vi "oax_GS Level Measurement.vi"(0 "scaled signals [EU]":waveform(dbl)[](array[waveform]), 5 "Start":dbl, 7 "Duration":dbl, 9 "select channel":u16, 11 "error in (no error)":errorcluster) -> (4 "Peak level [EU]":dbl, 6 "RMS level [EU]":dbl, 8 "vibration signals":waveform(dbl), 15 "error out":errorcluster)   [LabVIEW 2017]
uses:
  <vilib>/addons/Sound and Vibration/svt_Level/SVL Peak Level (1 Ch).vi
  <vilib>/addons/Sound and Vibration/svt_Level/SVL RMS Level (1 Ch).vi
  <vilib>/Waveform/WDTOps.llb/WDT Get Waveform Subset DBL (LV80).vi
  <vilib>/addons/Sound and Vibration/svt_Level/SoundVib_VibrationLevel.lvlib
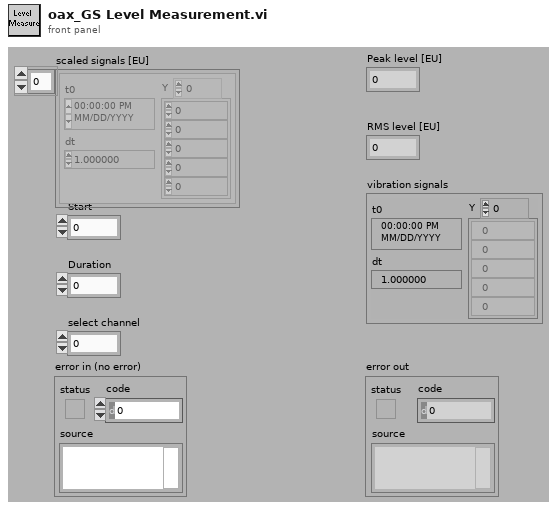
[diagram p1: front panel]
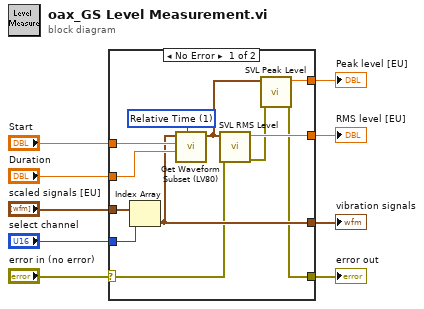
[diagram p0: block diagram]
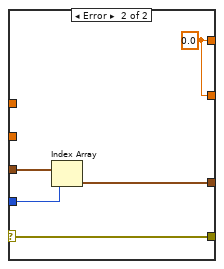
[diagram p2: hidden frame]
diagram:
  n1 = case shown="No Error" "error in (no error)" {
    selector: "error in (no error)" -> [w12 w26]
    tunnel: [w21 w25] -> w9
    tunnel: "Duration" -> [w19 _]
    tunnel: "Start" -> [w18 _]
    tunnel: [w16 w22] -> w6
    tunnel: [w15 w25] -> w5
    tunnel: "scaled signals [EU]" -> [w14 w24]
    tunnel: "select channel" -> [w13 w23]
    tunnel: [w10 w26] -> w1
    frame No Error {
      w17 = u16 1 items=["Index", "Relative Time"] ("Mode")
      n2 = Index Array(array=w14, index=w13) -> (element=w16:waveform(dbl))
      n3 = call-poly <vilib>:"Get Waveform Subset (LV80).vi"("start/duration format"=w17, "duration"=w19, "start samples/time"=w18, "waveform in"=w16) -> ("waveform out"=w20:waveform(dbl))  [unwired: 2 in, 3 out]
      n4 = call-poly <vilib>:"SVL RMS Level.vi"("error in (no error)"=w12, "scaled signal [EU]"=w20) -> ("error out"=w11:errorcluster, "RMS level [EU rms]"=w15:dbl)  [unwired: 7 in, 1 out]
      n5 = call-poly <vilib>:"SVL Peak Level.vi"("error in (no error)"=w11, "scaled signal [EU]"=w20) -> ("error out"=w10:errorcluster, "peak level [EU]"=w21:dbl)  [unwired: 7 in, 1 out]
    }
    frame Error {
      w25 = 0.0 ("peak level [EU]")
      n6 = Index Array(array=w24, index=w23) -> (element=w22:waveform(dbl))
    }
  }
  "Peak level [EU]" <- w9
  "vibration signals" <- w6
  "RMS level [EU]" <- w5
  "error out" <- w1
